vi "MKS946_Main.vi"(7 "stop_external":refnum<vi>, 8 "input cluster":T1) -> ()   [LabVIEW 2019]
doc: "Perform the acquisition. Replace the contents of this diagram with calls to acquisition hardware.\n_____\nBased on Delacor QMH Project Template 5.0.0.82."
uses:
  cluster_ref_MKS946.ctl
  MKS946_Global.vi
panel:
  out "P2T":dbl caption="Torr" format="%.2f"
  out "P1T":dbl caption="Torr" format="%.2f"
  out "status_log":bool caption="Status"
  out "Last Measurement":timestamp format="%<%Y-%m-%d %H:%M:%S>T"
  in  "stop":bool
  in  "Logging":bool=TRUE
  out "P2 Chart":waveform(dbl)[](graph)
  out "P1 Chart":waveform(dbl)[](graph)
  out "Status":bool
  in  "interval":dbl=5.0 caption="sec" format="%#_13g"
  out "P2":dbl caption="psig" format="%.2f"
  out "P1":dbl caption="psig" format="%.2f"
  in  "address":i32=253
  in  "visa_in":refnum<visa-resource-name>="COM28"
  # "MKS 946"
  # "Chart-Axis Control"
  # "QT Manifold"
  # "Root Exhaust"
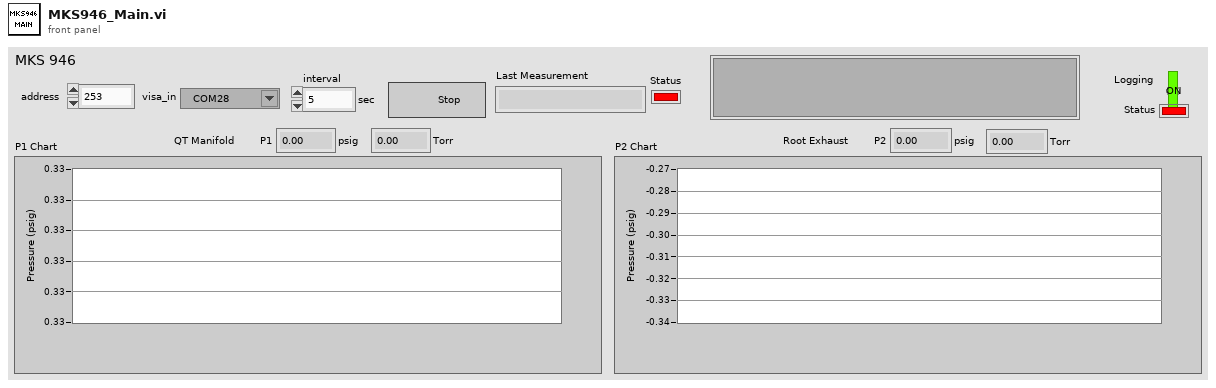
[diagram p1: front panel]
types:
  T1 = typedef "cluster_ref_MKS946.ctl" = cluster{"Status":refnum<vi>, "PR1":refnum<vi>, "PR2":refnum<vi>}
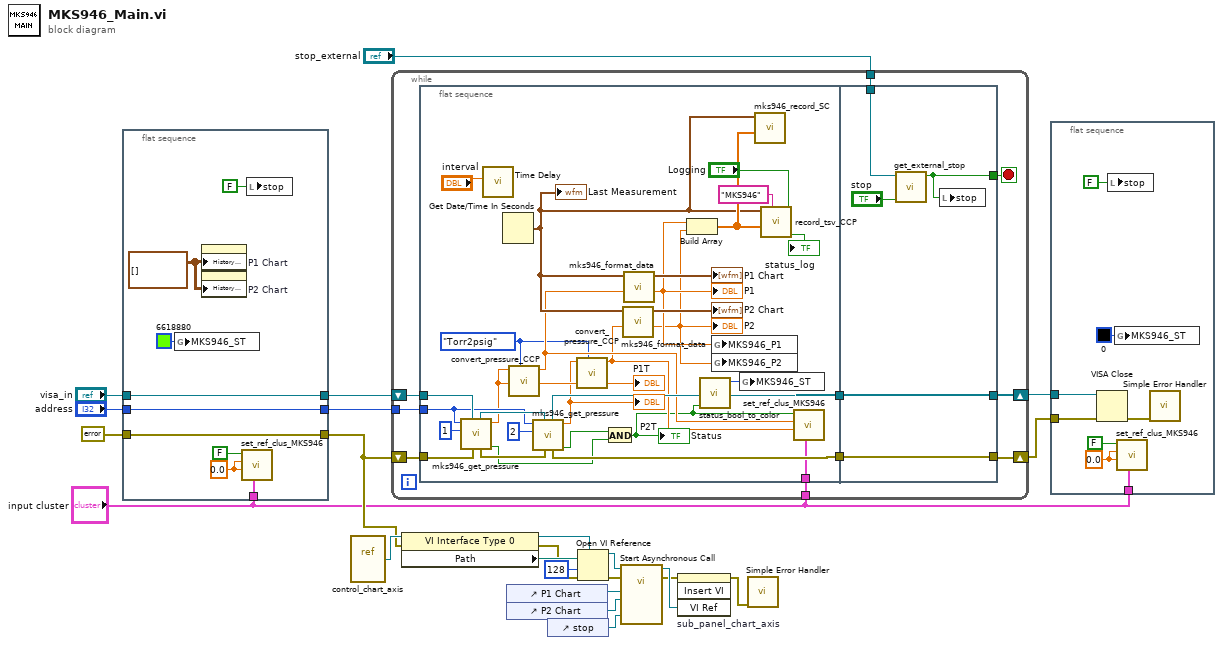
[diagram p0: block diagram]
diagram:
  n1 = flat-sequence {
    tunnel: "input cluster" -> [w32]
    tunnel: [w26] -> w6
    tunnel: [w29] -> w20
    tunnel: "address" -> [w29]
    tunnel: [w28] -> w18
    tunnel: "visa_in" -> [w28]
    tunnel: errorcluster {"status"=FALSE, "code"=0, "source"=""} ("error in") -> [w26]
    frame #0 {
      w27 = waveform(dbl)[][] [] ("History Data")
      w31 = 0.0 ("PR2")
      n2 = global write "MKS946_Global.vi" "MKS946_ST"(u32 6618880 ("MKS946_ST")) -> ()
      n3 = property on="P1 Chart" class="WFChart (strict)"("History Data"=w27) -> ()  [unwired: 2 in, 2 out]
      n4 = property on="P2 Chart" class="WFChart (strict)"("History Data"=w27) -> ()  [unwired: 2 in, 2 out]
      n5 = call "set_ref_clus_MKS946.vi"("cluster_ref"=w32, "PR2"=w31, "PR1"=w31, "status"=FALSE) -> ()  [unwired: 8 in]
      n6 = local write "stop"(FALSE ("stop")) -> ()
    }
  }
  n7 = vi-ref "control_chart_axis.vi"() -> (w12:refnum<vi>)
  n8 = while {
    tunnel: w20 -> [w39]
    shift-right: [w40] -> w22
    shift-left: w18 -> [w42]
    shift-right: [w38] -> w21
    shift-left: w6 -> [w41]
    tunnel: "input cluster" -> [w37]
    tunnel: "stop_external" -> [w34]
    stop <- w33 stop-if-true
    n9 = flat-sequence {
      tunnel: w42 -> [w71]
      tunnel: w41 -> [w69]
      tunnel: w39 -> [w64]
      tunnel: w37 -> [w59]
      tunnel: [w67] -> w36
      tunnel: [w63] -> w35
      tunnel: [w75] -> w38
      tunnel: [w76] -> w40
      tunnel: w36 -> [w76]
      tunnel: w35 -> [w75]
      tunnel: w34 -> [w73]
      tunnel: [w72] -> w33
      frame #0 {
        w49 = enum16{"None", "Torr2psig"}."Torr2psig" ("conv_type")
        n10 = call "mks946_get_pressure.vi"("err_in"=w69, "visa_in"=w71, "channel"=1, "address"=w64) -> ("status"=w60:bool, "value"=w48:dbl, "err_out"=w66:errorcluster, "visa_out"=w68:refnum<visa-resource-name>)  [unwired: 3 in, 1 out]
        "P1T" <- w48
        n11 = call "Time Delay"("Delay Time (s)"="interval") -> ()  [unwired: 10 in, 1 out]
        n12 = Get Date/Time In Seconds() -> (seconds since 1Jan1904=w52:timestamp)
        "Last Measurement" <- w52
        n13 = call "convert_pressure_CCP.vi"("conv_type"=w49, "P_in"=w48) -> ("P_out"=w51:dbl)  [unwired: 9 in]
        n14 = call "mks946_get_pressure.vi"("err_in"=w66, "visa_in"=w68, "channel"=2, "address"=w64) -> ("status"=w61:bool, "value"=w47:dbl, "err_out"=w63:errorcluster, "visa_out"=w67:refnum<visa-resource-name>)  [unwired: 3 in, 1 out]
        "P2T" <- w47
        n15 = call "convert_pressure_CCP.vi"("conv_type"=w49, "P_in"=w47) -> ("P_out"=w50:dbl)  [unwired: 9 in]
        n16 = And(x=w61, y=w60) -> (x .and. y?=w43:bool)
        "Status" <- w43
        n17 = call "mks946_format_data.vi"("value"=w50, "time"=w52) -> ("value_out"=w45:dbl, "waveform_array"=→"P2 Chart":waveform(dbl)[])  [unwired: 8 in]
        "P2" <- w45
        n18 = call "mks946_format_data.vi"("value"=w51, "time"=w52) -> ("value_out"=w46:dbl, "waveform_array"=→"P1 Chart":waveform(dbl)[])  [unwired: 8 in]
        "P1" <- w46
        n19 = Build Array(w46, w45) -> (w53:dbl[])
        n20 = call "status_bool_to_color.vi"("status_bool_4"=w43) -> ("status_color"=w44:u32)  [unwired: 10 in]
        n21 = global write "MKS946_Global.vi" "MKS946_P1"(w46) -> ()
        n22 = global write "MKS946_Global.vi" "MKS946_P2"(w45) -> ()
        n23 = global write "MKS946_Global.vi" "MKS946_ST"(w44) -> ()
        n24 = call "mks946_record_SC.vi"("value_array"=w53, "time"=w52) -> ()  [unwired: 9 in, 1 out]
        n25 = call "record_tsv_CCP.vi"("logging_on"="Logging", "folder_name"="MKS946", "value_array"=w53, "time"=w52) -> ("status"=→"status_log":bool)  [unwired: 6 in, 1 out]
        n26 = call "set_ref_clus_MKS946.vi"("cluster_ref"=w59, "PR2"=w50, "PR1"=w51, "status"=w43) -> ()  [unwired: 8 in]
      }
      frame #1 {
        n27 = call "get_external_stop.vi"("stop_internal"="stop", "ref_stop_external"=w73) -> ("stop_output"=w72:bool)  [unwired: 9 in]
        n28 = local write "stop"(w72) -> ()
      }
    }
  }
  n29 = property class="VI Interface Type 0"(reference=w12, error in=w6) -> (reference out=w9:refnum<vi>, error out=w5:errorcluster, "Path"=w13:path)
  n30 = control-ref of="P1 Chart"() -> (w7:refnum<vi>)
  n31 = control-ref of="P2 Chart"() -> (w8:refnum<vi>)
  n32 = control-ref of="stop"() -> (w15:refnum<vi>)
  n33 = Open VI Reference(type specifier VI Refnum (for type only)=w9, vi path=w13, options=128, error in (no error)=w5) -> (vi reference=w11:refnum<vi>, error out=w4:errorcluster)  [unwired: 2 in]
  n34 = call-by-ref "Start Asynchronous Call"(reference=w11, error in=w4, "stop"=w15, "chart_2"=w8, "chart_1"=w7) -> (reference out=w14:refnum<vi>, error out=w3:errorcluster)  [unwired: 9 in]
  n35 = invoke on="sub_panel_chart_axis" class="SubPnl" method="Insert VI"(error in=w3, "VI Ref"=w14) -> (error out=w2:errorcluster)  [unwired: 2 in, 3 out]
  n36 = call <vilib>:"Simple Error Handler.vi"("error in (no error)"=w2) -> ()  [unwired: 4 in, 5 out]
  n37 = flat-sequence {
    tunnel: w22 -> [w84]
    tunnel: w21 -> [w83]
    tunnel: "input cluster" -> [w79]
    frame #0 {
      w81 = 0.0 ("PR2")
      n38 = VISA Close(VISA resource name=w84, error in (no error)=w83) -> (error out=w82:errorcluster)
      n39 = local write "stop"(FALSE ("stop")) -> ()
      n40 = global write "MKS946_Global.vi" "MKS946_ST"(u32 0 ("MKS946_ST")) -> ()
      n41 = call "set_ref_clus_MKS946.vi"("cluster_ref"=w79, "PR2"=w81, "PR1"=w81, "status"=FALSE) -> ()  [unwired: 8 in]
      n42 = call <vilib>:"Simple Error Handler.vi"("error in (no error)"=w82) -> ()  [unwired: 4 in, 5 out]
    }
  }
